vi "Build PSP URL.vi"(8 "error in (no error)":errorcluster, 10 "IP Address":string, 11 "Channel Ref in":T1 format="%.0x") -> (0 "error out":errorcluster, 2 "Shared Variable URL":string, 3 "Channel Ref out":T1 format="%.0x")   [LabVIEW 2015, in "Shared Variable Custom Device.lvlib"]
uses:
  Shared Variable Custom Device.lvlib
  <vilib>/NI Veristand/Custom Device API/Custom Device Item Ref.ctl
  Shared Variable Globals.vi
  <vilib>/NI Veristand/Custom Device API/Custom Device API.lvlib
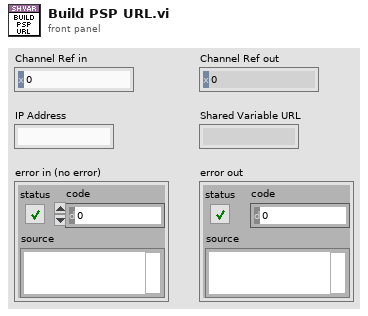
[diagram p1: front panel]
types:
  T1 = typedef "Custom Device API.lvlib/Custom Device Item Ref.ctl" = u64
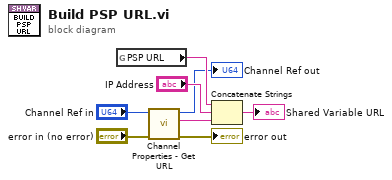
[diagram p0: block diagram]
diagram:
  n1 = global read "Shared Variable Globals.vi" "PSP URL"() -> (w8:string)
  n2 = call "Channel Properties - Get URL.vi"("error in (no error)"="error in (no error)", "Channel Ref in"="Channel Ref in") -> ("error out"=→"error out":errorcluster, "Shared Variable URL"=w7:string, "Channel Ref out"=→"Channel Ref out":T1)  [unwired: 7 in]
  n3 = Concatenate Strings(w8, "IP Address", w7) -> (→"Shared Variable URL":string)
